vi "Write Sub panel coin.vi"(8 "error in (no error)":errorcluster, 10 "Sub panel coin":refnum<vi>, 11 "USD ACTOR in":refnum<class "USD ACTOR.lvclass">) -> (0 "error out":errorcluster, 3 "USD ACTOR out":refnum<class "USD ACTOR.lvclass">)   [LabVIEW 2019, in "USD ACTOR.lvlib" / "USD ACTOR.lvclass"]
uses:
  USD ACTOR.lvclass
  USD ACTOR.lvclass/USD ACTOR.ctl
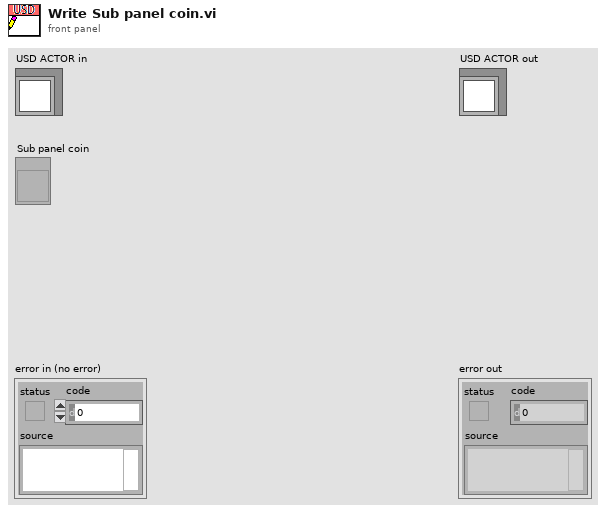
[diagram p1: front panel]
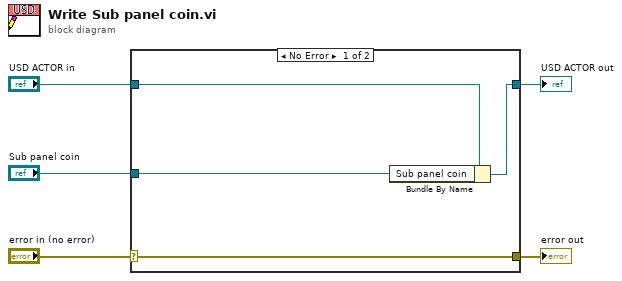
[diagram p0: block diagram]
diagram:
  n1 = case shown="No Error" "error in (no error)" {
    selector: "error in (no error)" -> [w9 w10]
    tunnel: [w9 w10] -> w4
    tunnel: [w7 w11] -> w2
    tunnel: "USD ACTOR in" -> [w8 w11]
    tunnel: "Sub panel coin" -> [w6 _]
    frame No Error {
      n2 = Bundle By Name(cluster=w8, "Sub panel coin"=w6) -> (w7:refnum<class "USD ACTOR.lvclass">)
    }
    frame Error {
    }
  }
  "error out" <- w4
  "USD ACTOR out" <- w2
